vi "Export File - Generate XML File.vi"(8 "error in (no error)":errorcluster, 10 "Target File":path=path "D:/Temp/UDP CD Test Files/XML Export/testExport.xml", 11 "Import/Export Data":T1 {"Tx Packets"."Tx Packet Data"."threadOptions"."pclDecimation" max=16 step=1; "Tx Packets"."Tx Packet Data"."threadOptions"."loopPeriod" max=16 step=1; "Tx Packets"."Tx Packet Data"."threadOptions"."targetPriority" min=-2 max=16 step=1; "Tx Packets"."Tx Packet Data"."threadOptions"."targetProcessor" min=-2 max=16 step=1; "Tx Packets"."Tx Packet Data"."Endianness" items=["big-endian"=0, "little-endian"=2]; "Rx Packets"."Rx Packet Data"."targetPriority" min=-2 max=16 step=1; "Rx Packets"."Rx Packet Data"."targetProcessor" min=-2 max=16 step=1; "Rx Packets"."Rx Packet Data"."Endianness" items=["big-endian"=0, "little-endian"=2]}) -> (0 "error out":errorcluster)   [LabVIEW 2019, in "UDP-Custom-Device System Explorer.lvlib"]
uses:
  UDP-Custom-Device System Explorer.lvlib
  Types/XML - New/ImpExp - Data.ctl
  Types/XML - New/ImpExp - Main Data.ctl
  <vilib>/NI VeriStand/Custom Device API/Custom Device Item Info.ctl
  Types/XML - New/ImpExp - Rx Packets Data.ctl
  Types/XML - New/ImpExp - Rx Packet Data.ctl
  Shared/Types/Shared - Channel Data Type.ctl
  Shared/Types/Shared - Buffered.PacketInfo.ctl
  Shared/Types/Shared - Pointer Encoding.ctl
  Shared/Types/Shared - Receive Buffer Options.ctl
  Shared/Types/Shared - Transmit Buffer Options.ctl
  Shared/Types/Shared - New Data Options.ctl
  Shared/Types/Shared - Thread Management.ctl
  Types/XML - New/ImpExp - Tx Packets Data.ctl
  Types/XML - New/ImpExp - Tx Packet Data.ctl
  Shared/Types/Shared - Transmit Flag Options.ctl
  Shared/Types/Shared - Transmit Echo Options.ctl
  Types/Threading/Thread Configuration.ctl
  Types/Threading/Thread Sync Reference.ctl
  System.Xml
  <vilib>/NI VeriStand/Custom Device API/Custom Device API.lvlib
  Shared/UDP-Custom-Device Shared.lvlib
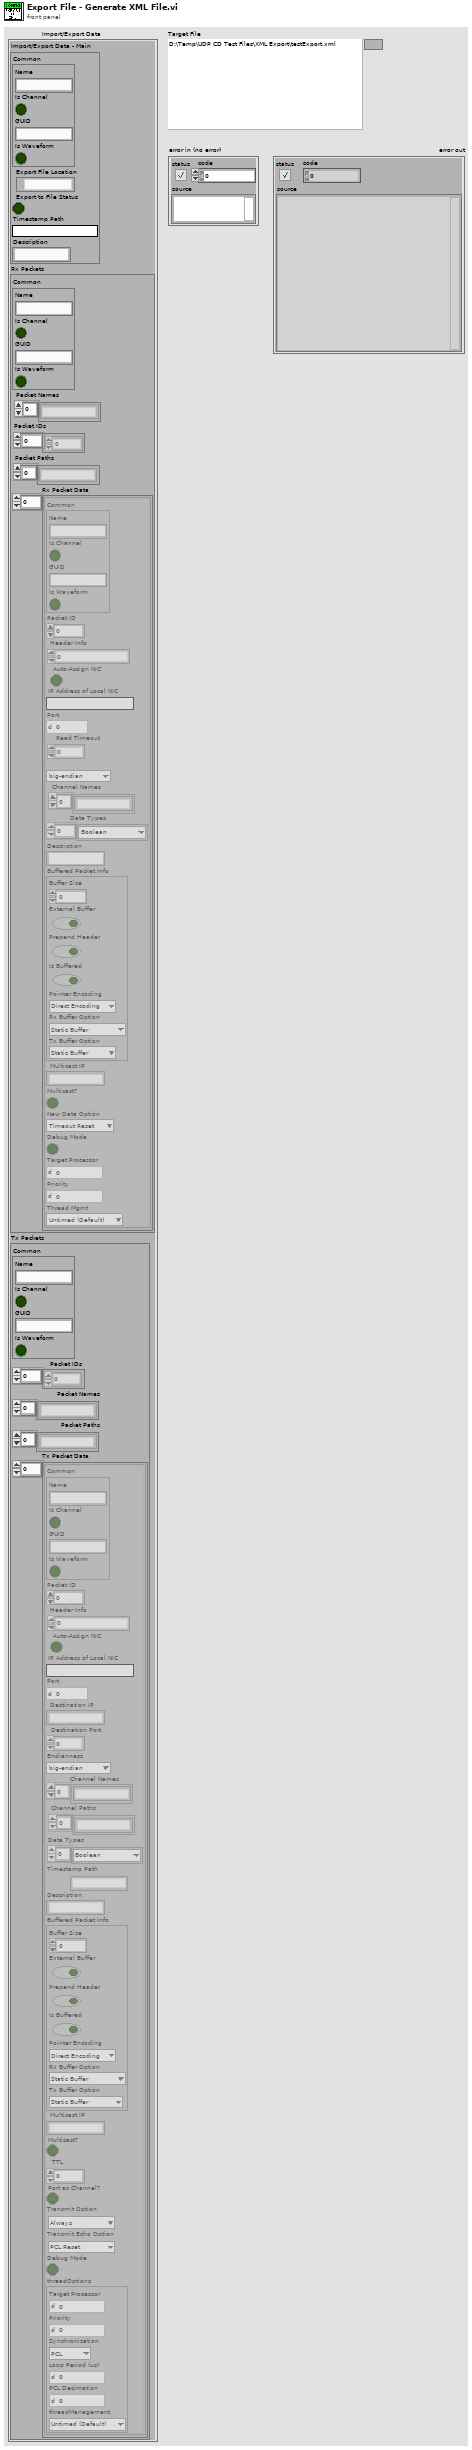
[diagram p1: front panel]
types:
  T1 = typedef "UDP-Custom-Device System Explorer.lvlib/ImpExp - Data.ctl" = cluster{"Import/Export Data - Main":T2, "Rx Packets":T4, "Tx Packets":T13}
  T2 = typedef "UDP-Custom-Device System Explorer.lvlib/ImpExp - Main Data.ctl" = cluster{"Common":T3, "Export File Location":path, "Export to File Status":bool, "Timestamp Path":string, "Description":string}
  T3 = typedef "Custom Device API.lvlib/Custom Device Item Info.ctl" = cluster{"Name":string, "Is Channel":bool, "GUID":string, "Is Waveform":bool}
  T4 = typedef "UDP-Custom-Device System Explorer.lvlib/ImpExp - Rx Packets Data.ctl" = cluster{"Common":T3, "Packet Names":string[], "Packet IDs":i32[], "Packet Paths":string[], "Rx Packet Data":T5[]}
  T5 = typedef "UDP-Custom-Device System Explorer.lvlib/ImpExp - Rx Packet Data.ctl" = cluster{"Common":T3, "Packet ID":i32, "Header Info":u32, "Auto-Assign NIC":bool, "IP Address of Local NIC":string, "Port":u16, "Read Timeout":i32, "Endianness":u16, "Channel Names":string[], "Data Types":T6[], "Description":string, "Buffered Packet Info":T7, "Multicast IP":string, "Multicast?":bool, "New Data Option":T11, "Debug Mode":bool, "targetProcessor":i8, "targetPriority":i16, "Thread Mgmt":T12}
  T6 = typedef "UDP-Custom-Device Shared.lvlib/Shared - Channel Data Type.ctl" = enum16{"Boolean", "Single", "Double", "I8", "I16", "I32", "I64", "U8", "U16", "U32", "U64"}
  T7 = typedef "UDP-Custom-Device Shared.lvlib/Shared - Buffered.PacketInfo.ctl" = cluster{"Buffer Size":i32, "External Buffer":bool, "Prepend Header":bool, "Is Buffered":bool, "Pointer Encoding":T8, "Rx Buffer Option":T9, "Tx Buffer Option":T10}
  T8 = typedef "UDP-Custom-Device Shared.lvlib/Shared - Pointer Encoding.ctl" = enum16{"Direct Encoding", "Conversion Encoding"}
  T9 = typedef "UDP-Custom-Device Shared.lvlib/Shared - Receive Buffer Options.ctl" = enum16{"Static Buffer", "Circular Buffer", "Circular Buffer + Size", "Internal Cache", "Internal Cache + Size", "Ping Pong", "Ping Pong + Size"}
  T10 = typedef "UDP-Custom-Device Shared.lvlib/Shared - Transmit Buffer Options.ctl" = enum16{"Static Buffer", "FIFO Buffer", "FIFO Buffer + Port"}
  T11 = typedef "UDP-Custom-Device Shared.lvlib/Shared - New Data Options.ctl" = enum16{"Timeout Reset", "Counter"}
  T12 = typedef "UDP-Custom-Device Shared.lvlib/Shared - Thread Management.ctl" = enum16{"Untimed (Default)", "Timed (High Priority)"}
  T13 = typedef "UDP-Custom-Device System Explorer.lvlib/ImpExp - Tx Packets Data.ctl" = cluster{"Common":T3, "Packet IDs":i32[], "Packet Names":string[], "Packet Paths":string[], "Tx Packet Data":T14[]}
  T14 = typedef "UDP-Custom-Device System Explorer.lvlib/ImpExp - Tx Packet Data.ctl" = cluster{"Common":T3, "Packet ID":i32, "Header Info":u32, "Auto-Assign NIC":bool, "IP Address of Local NIC":string, "Port":u16, "Destination IP":string, "Destination Port":u16, "Endianness":u16, "Channel Names":string[], "Channel Paths":string[], "Data Types":T6[], "Timestamp Path":string, "Description":string, "Buffered Packet Info":T7, "Multicast IP":string, "Multicast?":bool, "TTL":u16, "Port as Channel?":bool, "Transmit Option":T15, "Transmit Echo Option":T16, "Debug Mode":bool, "threadOptions":T17}
  T15 = typedef "UDP-Custom-Device Shared.lvlib/Shared - Transmit Flag Options.ctl" = enum16{"Always", "One-Shot", "Toggle"}
  T16 = typedef "UDP-Custom-Device Shared.lvlib/Shared - Transmit Echo Options.ctl" = enum16{"PCL Reset", "Counter", "Mirror"}
  T17 = typedef "UDP-Custom-Device System Explorer.lvlib/Thread Configuration.ctl" = cluster{"targetProcessor":i8, "targetPriority":i16, "Synchronization":T18, "loopPeriod":u32, "pclDecimation":u16, "threadManagement":T12}
  T18 = typedef "UDP-Custom-Device System Explorer.lvlib/Thread Sync Reference.ctl" = enum16{"PCL", "Async"}
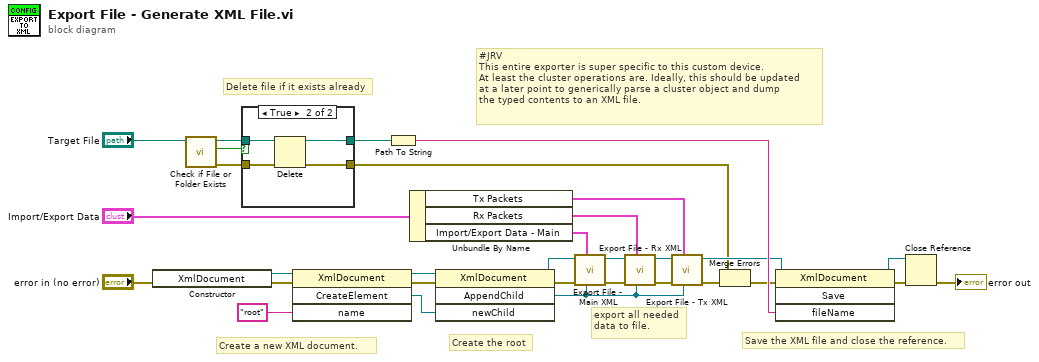
[diagram p0: block diagram]
diagram:
  # "#JRV\nThis entire exporter is super specific to this custom device.\nAt least the cluster operations are. Ideally, this should be updated\nat a later point to generically parse a cluster object and dump\nthe typed contents to an XML file."
  # "Save the XML file and close the reference."
  # "export all needed\ndata to file."
  # "Create the root"
  # "Create a new XML document."
  # "Delete file if it exists already"
  n1 = constructor class="XmlDocument"(error in="error in (no error)") -> (reference out=w23:refnum<k24>, error out=w22:errorcluster)  [unwired: 2 in, 1 out]
  n2 = call <vilib>:"Check if File or Folder Exists.vi"("path"="Target File") -> ("error out"=w4:errorcluster, "file or folder exists?"=w7:bool, "dup path"=w6:path)  [unwired: 8 in]
  n3 = case shown="True" w7 {
    tunnel: w6 -> [w32 w37]
    tunnel: [w32 w36] -> w5
    tunnel: w4 -> [w33 w35]
    tunnel: [w33 w34] -> w1
    frame False {
    }
    frame True {
      n4 = Delete(path (use dialog)=w37, error in=w35) -> (deleted path=w36:path, error out=w34:errorcluster)  [unwired: 3 in, 1 out]
    }
  }
  n5 = invoke class="XmlDocument" method="CreateElement"(reference=w23, error in=w22, "name"="root" ("Tag Name")) -> (reference out=w20:refnum<k24>, error out=w18:errorcluster, "CreateElement"=w21:refnum<k24>)  [unwired: 1 in, 1 out]
  n6 = Path To String(path=w5) -> (string=w28:string)
  n7 = Unbundle By Name("Import/Export Data") -> ("Tx Packets"=w11:T13, "Rx Packets"=w14:T4, "Import/Export Data - Main"=w30:T2)
  n8 = invoke class="XmlDocument" method="AppendChild"(reference=w20, error in=w18, "newChild"=w21) -> (reference out=w19:refnum<k24>, error out=w17:errorcluster, "AppendChild"=w9:refnum<k24>)  [unwired: 1 in, 1 out]
  n9 = call "Export File - Main XML.vi"("RootNode"=w9, "Import/Export Data - Main"=w30, "error in (no error)"=w17, "XmlDocument in"=w19) -> ("error out"=w16:errorcluster, "XmlDocument out"=w15:refnum<k24>)  [unwired: 6 in]
  n10 = call "Export File - Rx XML.vi"("RootNode"=w9, "Rx Packets"=w14, "error in (no error)"=w16, "XmlDocument in"=w15) -> ("error out"=w10:errorcluster, "XmlDocument out"=w13:refnum<k24>)  [unwired: 6 in]
  n11 = call "Export File - Tx XML.vi"("RootNode"=w9, "Tx Packets"=w11, "error in (no error)"=w10, "XmlDocument in"=w13) -> ("error out"=w3:errorcluster, "XmlDocument out"=w12:refnum<k24>)  [unwired: 6 in]
  n12 = Merge Errors(w1, w3) -> (w2:errorcluster)
  n13 = invoke class="XmlDocument" method="Save"(reference=w12, error in=w2, "fileName"=w28) -> (reference out=w27:refnum<k24>, error out=w26:errorcluster)  [unwired: 1 in, 2 out]
  n14 = Close Reference(reference=w27, error in (no error)=w26) -> (error out=→"error out":errorcluster)
